vi "Caraya Time Measurement Runner.vi"() -> ()   [LabVIEW 2018]
uses:
  Common Support/Common Support.lvlib
panel:
  in  "Calculate Temperature Change":bool=TRUE
  in  "Thermal Chamber Response Simulator_Init":bool=TRUE
  in  "Get Chamber Status":bool=TRUE
  in  "GUI Interlock Tester":bool=TRUE
  in  "Convert Shutdown Furnace to Heater State Enum":bool=TRUE
  in  "Action Update Ramp Rate":bool=TRUE
  in  "Action Update Set Point":bool=TRUE
  in  "Action Update Heater State":bool=TRUE
  in  "All Test":bool
  out "Caraya In Progress":bool
  out "Caraya report":string
  out "Caraya Testing time (seconds)":dbl
  in  "Multiplier of runs":i32=10
  out "No. of Tests":i32=10
  # "If \"All Test\" is true, then all of selected and unselected tests \nbelow will be executed and each test will be executed only \nonce independently of \"Multiplier of runs\"."
  # "Caraya"
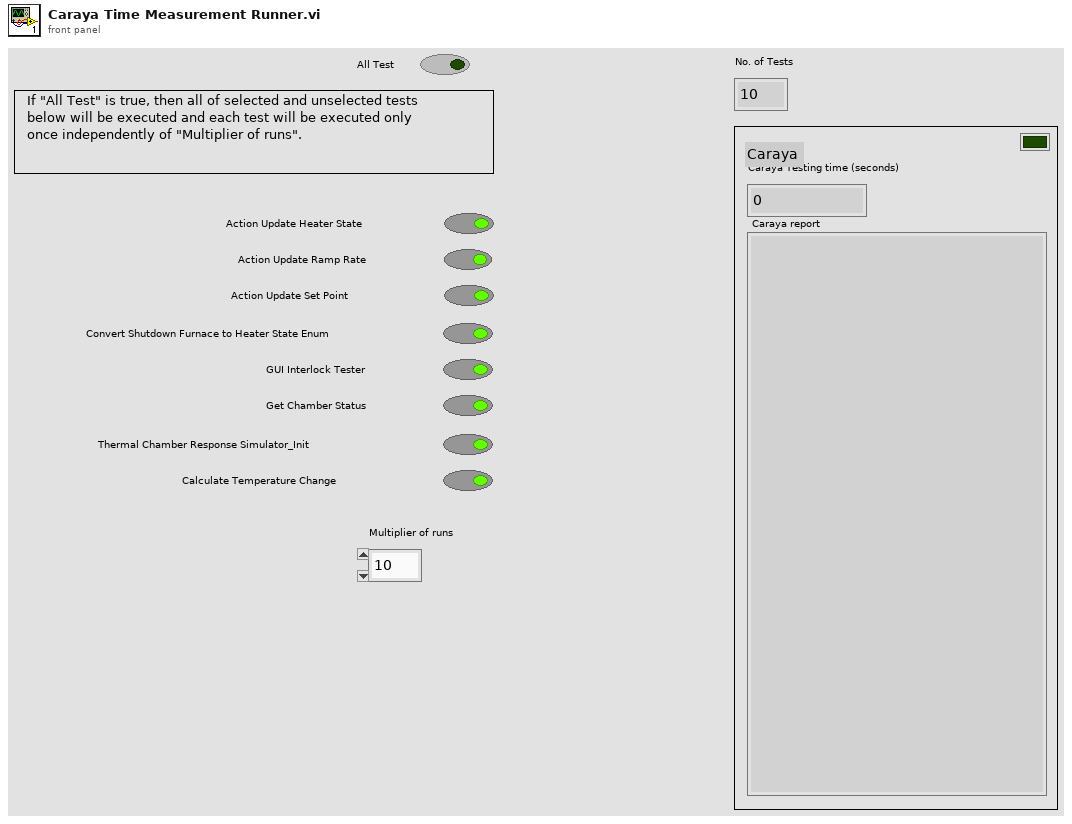
[diagram p1: front panel]
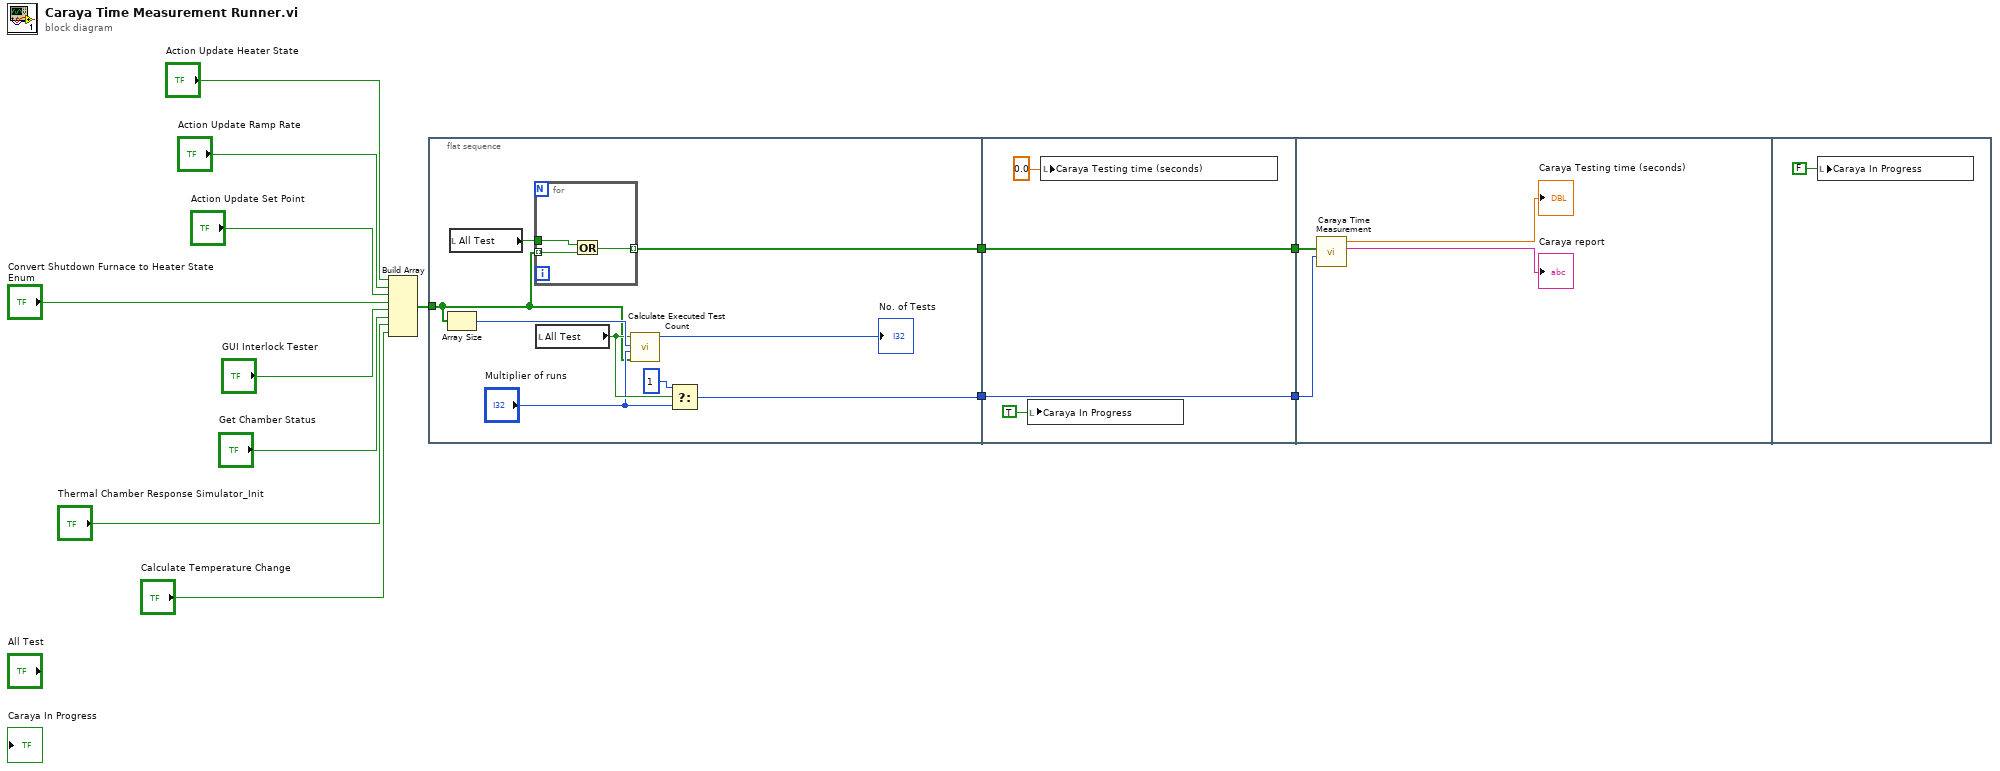
[diagram p0: block diagram]
diagram:
  n1 = Build Array("Action Update Heater State", "Action Update Ramp Rate", "Action Update Set Point", "Convert Shutdown Furnace to Heater State Enum", "GUI Interlock Tester", "Get Chamber Status", "Thermal Chamber Response Simulator_Init", "Calculate Temperature Change") -> (w8:bool[])
  n2 = flat-sequence {
    tunnel: [w18] -> w11
    tunnel: w8 -> [w16]
    tunnel: [w15] -> w5
    tunnel: [w28] -> w13
    tunnel: [w27] -> w12
    tunnel: w11 -> [w27]
    tunnel: w5 -> [w28]
    tunnel: w13 -> [w31]
    tunnel: w12 -> [w30]
    frame #0 {
      n3 = Array Size(array=w16) -> (size(s)=w22:i32)
      n4 = local read "All Test"() -> (w14:bool)
      n5 = for {
        tunnel: w16 -> [w25] mode=indexing
        tunnel: [w23] -> w15 mode=indexing
        tunnel: w14 -> [w24]
        n6 = Or(x=w24, y=w25) -> (x .or. y?=w23:bool)
      }
      n7 = local read "All Test"() -> (w20:bool)
      n8 = call "Calculate Executed Test Count.vi"("Test Selector Array"=w16, "Multiplier of Runs"="Multiplier of runs", "All Test Count"=w22, "Run All Tests"=w20) -> ("Executed Test Count"=→"No. of Tests":i32)  [unwired: 7 in]
      n9 = Select(t=1, s=w20, f="Multiplier of runs") -> (s? t:f=w18:i32)
    }
    frame #1 {
      n10 = local write "Caraya In Progress"(TRUE) -> ()
      n11 = local write "Caraya Testing time (seconds)"(0.0) -> ()
    }
    frame #2 {
      n12 = call "Caraya Time Measurement.vi"("No. of Runs"=w30, "Test Cases"=w31) -> ("Caraya report"=→"Caraya report":string, "ICov Testing time (seconds)"=→"Caraya Testing time (seconds)":dbl)  [unwired: 8 in]
    }
    frame #3 {
      n13 = local write "Caraya In Progress"(FALSE) -> ()
    }
  }
